vi "Continuous data for enqueue.vi"(8 "error in (no error)":errorcluster, 10 "Input Data":dbl[](array[numeric]), 11 "Target number of points (per frame)":u32) -> (0 "error out":errorcluster, 1 "Full Frame Data":dbl[](array[numeric]), 2 "Remaining Data":dbl[](array[numeric]), 3 "Total number of points acquired":i32)   [LabVIEW 2017]
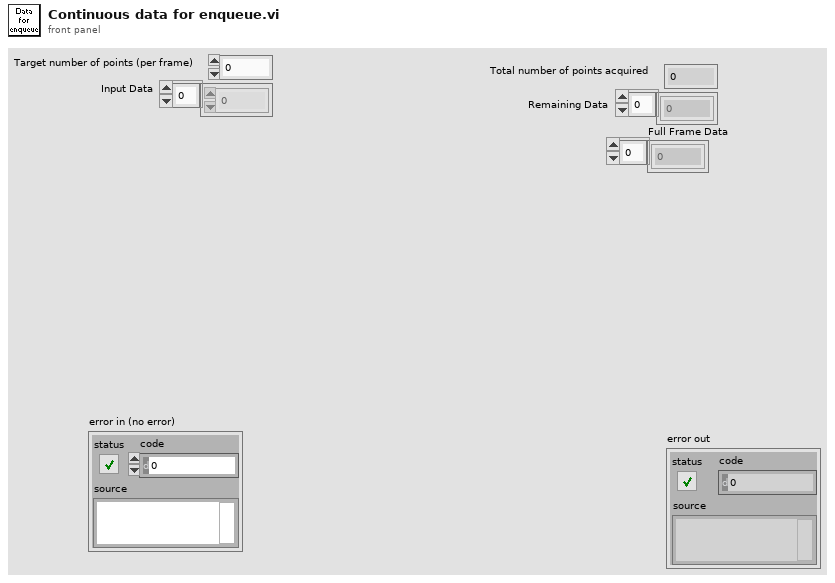
[diagram p1: front panel]
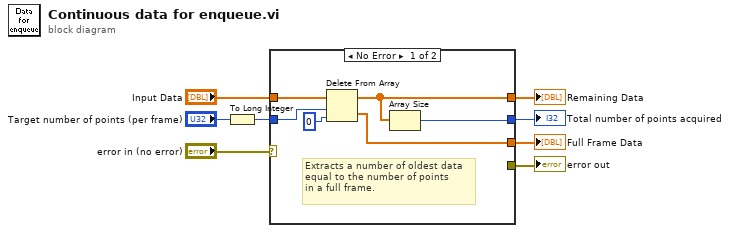
[diagram p0: block diagram]
diagram:
  n1 = To Long Integer(number="Target number of points (per frame)") -> (32bit integer=w1:i32)
  n2 = case shown="No Error" "error in (no error)" {
    selector: "error in (no error)" -> [_ w15]
    tunnel: "Input Data" -> [w11 w17]
    tunnel: w1 -> [w9 w16]
    tunnel: [w12 w17] -> w6
    tunnel: [w13 w16] -> w5
    tunnel: [_ w15] -> w4
    tunnel: [w14 _] -> w3
    frame No Error {
      # "Extracts a number of oldest data\nequal to the number of points\nin a full frame."
      n3 = Delete From Array "Delete From Array"(array=w11, length=w9, index=0) -> (deleted portion=w14:dbl[], array with subset deleted=w12:dbl[])
      n4 = Array Size(array=w12) -> (size(s)=w13:i32)
    }
    frame Error {
    }
  }
  "error out" <- w4
  "Total number of points acquired" <- w5
  "Remaining Data" <- w6
  "Full Frame Data" <- w3
